vi "Global_Settings.vi"(7 "Enum":T3, 8 "error in":errorcluster, 9 "Design Constants In":T1={"P_amb (psia)"=14.7, "T_in (Deg F)"=530.0, "R_air (ft*lbf)/(lbm*R)"=53.35, "g_c (lbm*ft)/(lbf*s^2)"=32.17, "specific heat ratio"=1.4, "Viscousity (lbm)/(ft*s)"=1.21e-05, "Cd"=0.61, "Mass Flow (lbm/min) vs. Pressure Drop (inH2O) - Real Data"=[[0.5, 0.0149], [1.0, 0.0619], [1.5, 0.139], [2.0, 0.249], [2.5, 0.385], [3.5, 0.73]]} {"Mass Flow (lbm/min) vs. Pressure Drop (inH2O) - Real Data" format="%_3g"; "P_amb (psia)" format="%#_4g"}, 10 "Design Tuners In":T2 {"OAR" items=["0.92"=0.92, "0.93"=0.93, "0.94"=0.94, "0.95"=0.95, "0.96"=0.96]; "D_h (in)" items=["0.0625"=0.0625, "0.125"=0.125, "0.250"=0.25]; "Pipe_Diameter (in)" min=0.1 max=6.0 scale=0.0..6.0 scale format="%#_3g"; "Length (in)" min=0.1 max=5.0 scale=0.0..6.0 scale format="%#_3g"; "Outlet Diameter (in)" min=0.1 max=5.0 scale=0.0..5.0 scale format="%#_3g"; "Inlet Diameter (in)" min=0.1 max=5.0 scale=0.0..5.0}) -> (0 "error out":errorcluster, 1 "Design Tuners Out":T2={"Inlet Diameter (in)"=0.1, "Outlet Diameter (in)"=0.1, "Length (in)"=0.1, "Pipe_Diameter (in)"=0.1, "D_h (in)"=0.125, "OAR"=0.95, "Run Optimizer"=FALSE} {"OAR" items=["0.92"=0.92, "0.93"=0.93, "0.94"=0.94, "0.95"=0.95, "0.96"=0.96]; "D_h (in)" items=["0.0625"=0.0625, "0.125"=0.125, "0.250"=0.25]; "Pipe_Diameter (in)" min=0.1 max=6.0 scale=0.0..6.0 scale format="%#_3g"; "Length (in)" min=0.1 max=5.0 scale=0.0..6.0 scale format="%#_3g"; "Outlet Diameter (in)" min=0.1 max=5.0 scale=0.0..5.0 scale format="%#_3g"; "Inlet Diameter (in)" min=0.1 max=5.0 scale=0.0..5.0}, 2 "Design Constants Out":T1={"P_amb (psia)"=14.7, "T_in (Deg F)"=70.0, "R_air (ft*lbf)/(lbm*R)"=53.35, "g_c (lbm*ft)/(lbf*s^2)"=32.17, "specific heat ratio"=1.4, "Viscousity (lbm)/(ft*s)"=1.21e-05, "Cd"=0.61, "Mass Flow (lbm/min) vs. Pressure Drop (inH2O) - Real Data"=[[0.5, 0.015], [1.0, 0.062], [1.5, 0.141], [2.0, 0.252], [2.5, 0.395], [3.5, 0.778]]} {"Mass Flow (lbm/min) vs. Pressure Drop (inH2O) - Real Data" format="%_3g"; "P_amb (psia)" format="%#_4g"})   [LabVIEW 2025]
uses:
  controls/Get_Set_Enum.ctl
  controls/Tuners.ctl
  controls/Constants.ctl
panel:
  # "Empirical Flow Path Data"
  # "Mass Flow\n (lbm/min)"
  # "Pressure Drop \n    (inH2O)"
  # "Empirical Flow Path Data"
  # "Mass Flow\n (lbm/min)"
  # "Pressure Drop \n    (inH2O)"
  # "Honeycomb Parameters"
  # "Orifice Parameters"
  # "Pipe Parameters"
  # "AIRFLOW SIMULATOR"
  # "Mass_flowrate"
  # "Pipe_Diameter"
  # "Outlet_Diameter"
  # "Inlet_Diameter"
  # "Honeycomb_Length"
  # "Honeycomb Parameters"
  # "Orifice Parameters"
  # "Pipe Parameters"
  # "AIRFLOW SIMULATOR"
  # "Mass_flowrate"
  # "Pipe_Diameter"
  # "Outlet_Diameter"
  # "Inlet_Diameter"
  # "Honeycomb_Length"
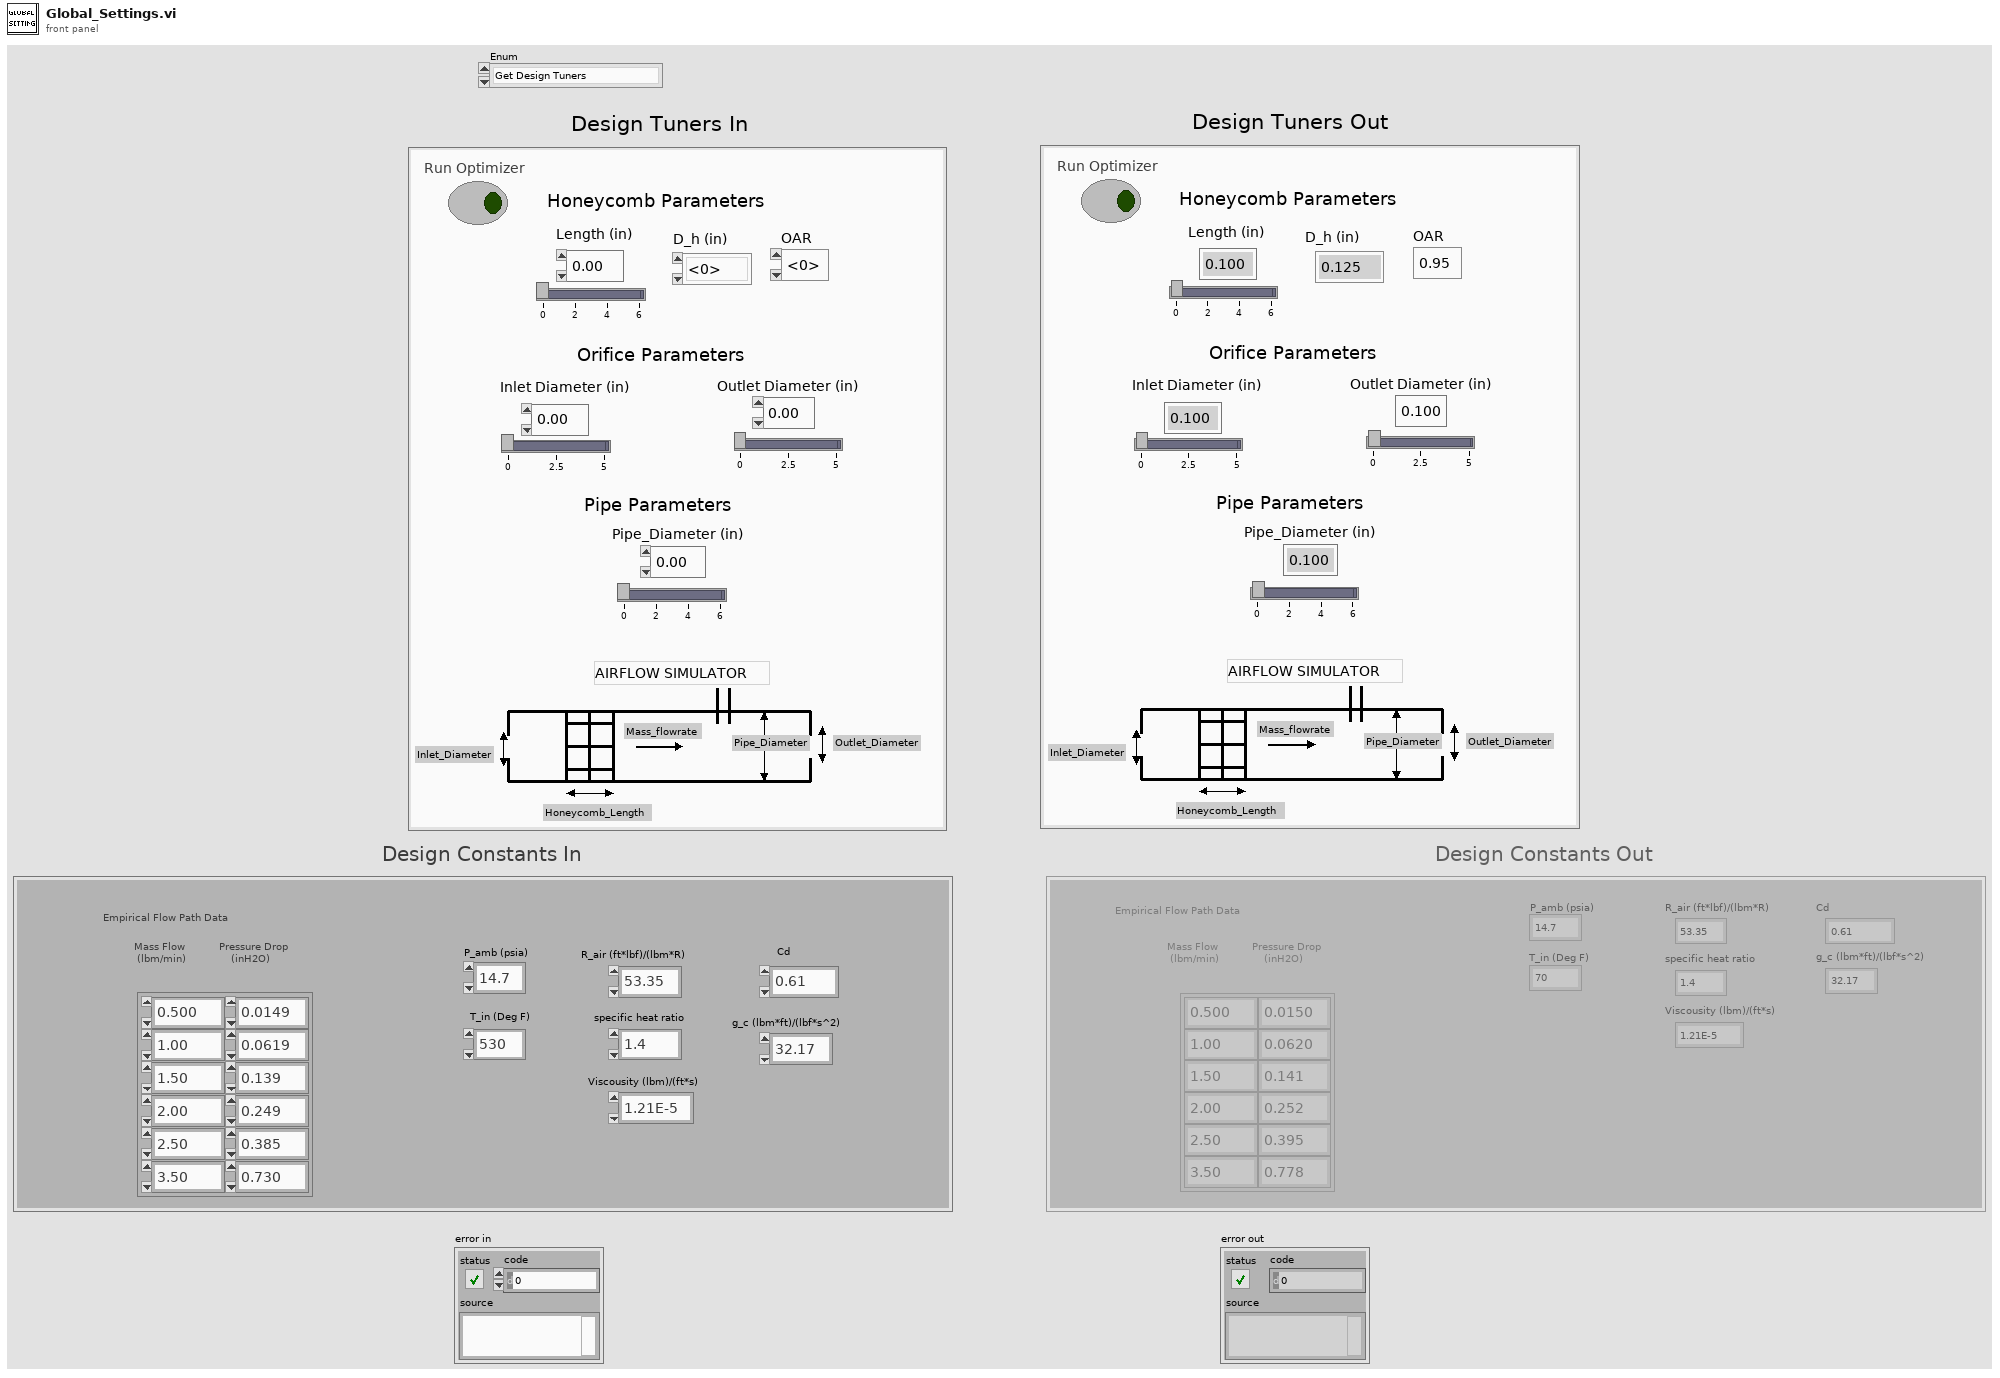
[diagram p1: front panel]
types:
  T1 = typedef "Constants.ctl" = cluster{"P_amb (psia)":dbl, "T_in (Deg F)":dbl, "R_air (ft*lbf)/(lbm*R)":dbl, "g_c (lbm*ft)/(lbf*s^2)":dbl, "specific heat ratio":dbl, "Viscousity (lbm)/(ft*s)":dbl, "Cd":dbl, "Mass Flow (lbm/min) vs. Pressure Drop (inH2O) - Real Data":dbl[][]}
  T2 = typedef "Tuners.ctl" = cluster{"Inlet Diameter (in)":dbl, "Outlet Diameter (in)":dbl, "Length (in)":dbl, "Pipe_Diameter (in)":dbl, "D_h (in)":dbl, "OAR":dbl, "Run Optimizer":bool}
  T3 = typedef "Get_Set_Enum.ctl" = enum16{"Get Design Tuners", "Set Design Tuners", "Get Design Constants", "Set Design Constants"}
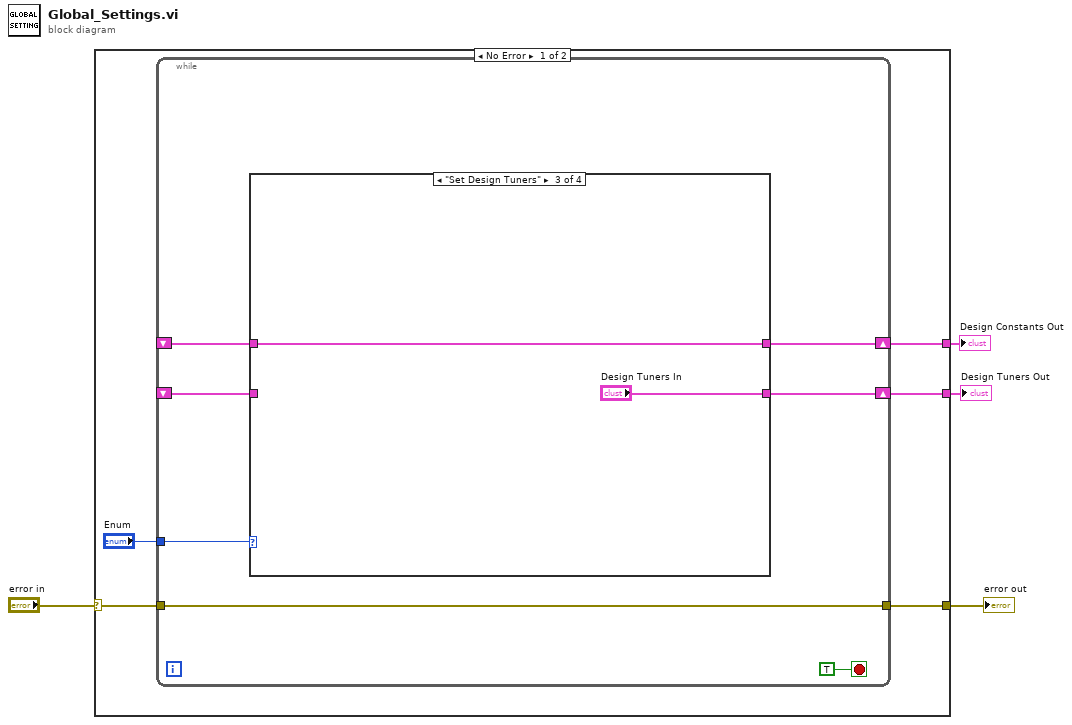
[diagram p0: block diagram]
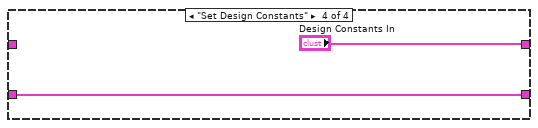
[diagram p4: hidden frame]
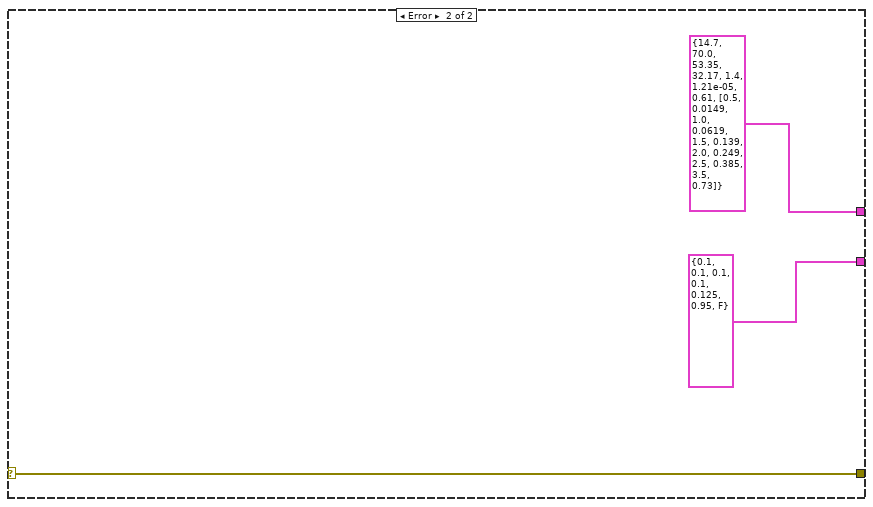
[diagram p5: hidden frame]
diagram:
  n1 = case shown="No Error" "error in" {
    selector: "error in" -> [w6 w27]
    tunnel: [w8 T1 {"P_amb (psia)"=14.7, "T_in (Deg F)"=70.0, "R_air (ft*lbf)/(lbm*R)"=53.35, "g_c (lbm*ft)/(lbf*s^2)"=32.17, "specific heat ratio"=1.4, "Viscousity (lbm)/(ft*s)"=1.21e-05, "Cd"=0.61, "Mass Flow (lbm/min) vs. Pressure Drop (inH2O) - Real Data"=[[0.5, 0.0149], [1.0, 0.0619], [1.5, 0.139], [2.0, 0.249], [2.5, 0.385], [3.5, 0.73]]} ("Design Constants In")] -> w2
    tunnel: [w7 w27] -> w3
    tunnel: [w5 T2 {"Inlet Diameter (in)"=0.1, "Outlet Diameter (in)"=0.1, "Length (in)"=0.1, "Pipe_Diameter (in)"=0.1, "D_h (in)"=0.125, "OAR"=0.95, "Run Optimizer"=FALSE} ("Tuners In")] -> w1
    frame No Error {
      n2 = while {
        tunnel: "Enum" -> [w16]
        shift-right: [w13] -> w8
        shift-left: _ -> [w14]
        tunnel: [w12] -> w7
        tunnel: w6 -> [w12]
        shift-right: [w11] -> w5
        shift-left: _ -> [w10]
        stop <- TRUE stop-if-true
        n3 = case shown="\"Set Design Tuners\"" w16 {
          tunnel: w14 -> [w18 w20 w21 _]
          tunnel: [w18 w20 w21 "Design Constants In"] -> w13
          tunnel: [w17 w19 "Design Tuners In" w23] -> w11
          tunnel: w10 -> [w17 w19 _ w23]
          frame "Get Design Tuners", Default {
          }
          frame "Get Design Constants" {
          }
          frame "Set Design Tuners" {
          }
          frame "Set Design Constants" {
          }
        }
      }
    }
    frame Error {
    }
  }
  "error out" <- w3
  "Design Constants Out" <- w2
  "Design Tuners Out" <- w1
